vi "Run Bfr Rx - Sized Handle Rollover.vi"(4 "Data Buffer":u64, 6 "Rollover Occurred?":bool, 7 "Size Offset in":u64, 8 "error in (no error)":errorcluster, 9 "Data Size (I32)":i32, 10 "Null Offset in":u64, 11 "Data Offset in":u64) -> (0 "error out":errorcluster, 2 "Null Offset out":u64, 3 "Data Offset out":u64, 5 "Size Offset out":u64)   [LabVIEW 2016, in "UDP-Custom-Device Engine.lvlib"]
uses:
  UDP-Custom-Device Engine.lvlib
  <vilib>/NI Veristand/VeriStand Data/Pointer Operations/Pointer.Write (I32).vi
  <vilib>/NI Veristand/VeriStand Data/VeriStand Data.lvlib
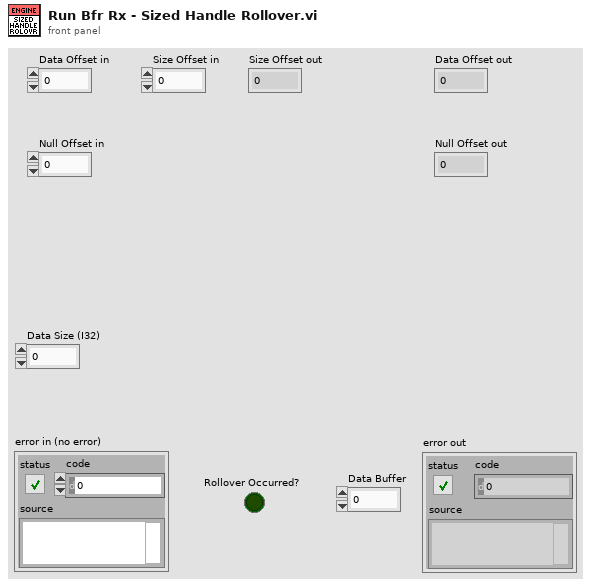
[diagram p1: front panel]
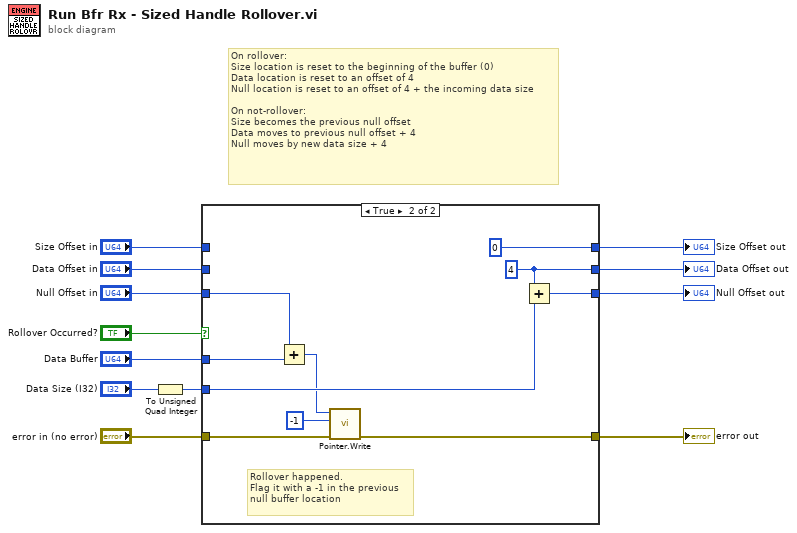
[diagram p0: block diagram]
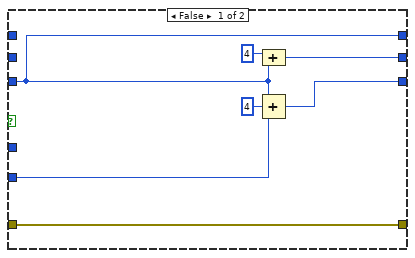
[diagram p2: hidden frame]
diagram:
  # "On rollover:\nSize location is reset to the beginning of the buffer (0)\nData location is reset to an offset of 4\nNull location is reset to an offset of 4 + the incoming data size\n\nOn not-rollover:\nSize becomes the previous null offset\nData moves to previous null offset + 4\nNull moves by new data size + 4"
  n1 = To Unsigned Quad Integer(1:"Data Size (I32)") -> (0:w10:u64)
  n2 = case shown="True" "Rollover Occurred?" {
    tunnel: w10 -> [w15 w26]
    tunnel: "error in (no error)" -> [w19 w21]
    tunnel: "Data Buffer" -> [_ w29]
    tunnel: "Null Offset in" -> [w14 w28]
    tunnel: "Size Offset in" -> [_ _]
    tunnel: "Data Offset in" -> [_ _]
    tunnel: [w14 u64 0] -> w4
    tunnel: [w17 w25] -> w3
    tunnel: [w13 w24] -> w2
    tunnel: [w19 w20] -> w1
    frame False {
      n3 = Compound Arithmetic op=ADD(u64 4 ("value"), w14) -> (w17:u64)
      n4 = Compound Arithmetic op=ADD(w14, u64 4 ("value"), w15) -> (w13:u64)
    }
    frame True {
      w25 = u64 4
      # "Rollover happened.\nFlag it with a -1 in the previous\nnull buffer location"
      n5 = Add(x=w28, y=w29) -> (x+y=w23:u64)
      n6 = call-poly <vilib>:"Pointer.Write.vi"("error in (no error)"=w21, "value"=-1, "pointer in"=w23) -> ("error out"=w20:errorcluster)  [unwired: 6 in, 2 out]
      n7 = Add(x=w25, y=w26) -> (x+y=w24:u64)
    }
  }
  "error out" <- w1
  "Null Offset out" <- w2
  "Data Offset out" <- w3
  "Size Offset out" <- w4
